vi "SubVI_Example_Eeprom.vi"(0 ".NET (Reference)":refnum<k24>, 5 "Write Flag":bool, 7 "Input Data":string, 9 "Starting Address":i32, 11 "Error In":errorcluster) -> (4 "Eeprom Data":string, 15 "Error Out":errorcluster)   [LabVIEW 2010]
uses:
  C:/Program Files (x86)/National Instruments/LabVIEW 2016/instr.lib/IDS/ueye.NET/uEyeDotNet.dll
  Program Files (x86)/National Instruments/LabVIEW 2016/instr.lib/IDS/ueye.NET/uEyeDotNet.dll
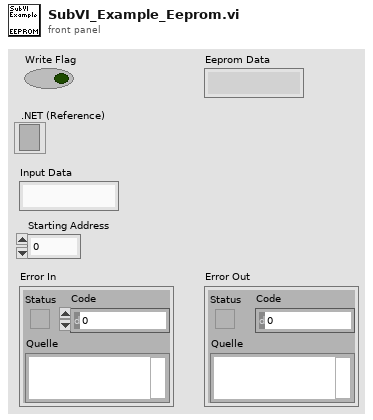
[diagram p1: front panel]
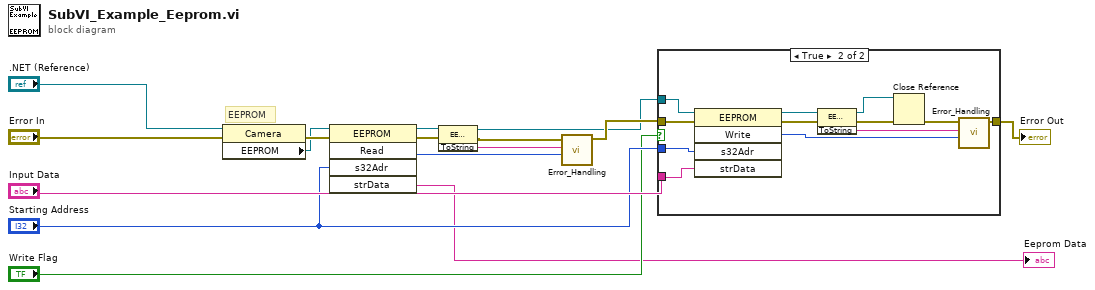
[diagram p0: block diagram]
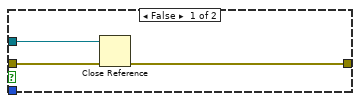
[diagram p2: hidden frame]
diagram:
  # "EEPROM"
  n1 = property on="Eigenschaftsknoten" class="Camera"(reference=".NET (Reference)", error in="Error In") -> (error out=w9:errorcluster, "EEPROM"=w8:refnum<k24>)  [unwired: 1 out]
  n2 = invoke class="EEPROM" method="Read"(reference=w8, error in=w9, "s32Adr"="Starting Address") -> (reference out=w13:refnum<k24>, error out=w14:errorcluster, "Read"=w15:i32, "strData"=→"Eeprom Data":string)  [unwired: 2 in, 1 out]
  n3 = invoke class="EEPROM" method="ToString"(reference=w13, error in=w14) -> (reference out=w1:refnum<k24>, error out=w2:errorcluster, "ToString"=w12:string)  [unwired: 1 in]
  n4 = call "Error_Handling.vi"("Error Code"=w15, "Error String"=w12, "Error In"=w2) -> ("Error Out"=w16:errorcluster)  [unwired: 8 in]
  n5 = case shown="True" "Write Flag" {
    tunnel: w1 -> [w17 w31]
    tunnel: "Starting Address" -> [_ w30]
    tunnel: w16 -> [w19 w29]
    tunnel: [w18 w23] -> w11
    tunnel: "Input Data" -> [_ w28]
    frame False {
      n6 = Close Reference(reference=w17, error in (no error)=w19) -> (error out=w18:errorcluster)
    }
    frame True {
      n7 = invoke class="EEPROM" method="Write"(reference=w31, error in=w29, "s32Adr"=w30, "strData"=w28) -> (reference out=w26:refnum<k24>, error out=w25:errorcluster, "Write"=w24:i32)  [unwired: 1 in, 2 out]
      n8 = invoke class="EEPROM" method="ToString"(reference=w26, error in=w25) -> (reference out=w20:refnum<k24>, error out=w22:errorcluster, "ToString"=w27:string)  [unwired: 1 in]
      n9 = Close Reference(reference=w20, error in (no error)=w22) -> (error out=w21:errorcluster)
      n10 = call "Error_Handling.vi"("Error Code"=w24, "Error String"=w27, "Error In"=w21) -> ("Error Out"=w23:errorcluster)  [unwired: 8 in]
    }
  }
  "Error Out" <- w11
